vi "Read Joystick.vi"(8 "Joystick Deadbanded Value (default of 0.1)":dbl, 11 "Joystick L 1 DevRef":T1) -> (1 "Joystick R 2 X Axis":dbl, 2 "Joystick L 1 Y Axis":dbl, 3 "Joystick L 1 X Axis":dbl)   [LabVIEW 2014]
uses:
  <vilib>/Rock Robotics/WPI/Joystick/WPI_JoystickDevRef.ctl
  <vilib>/Rock Robotics/WPI/Joystick/WPI_JoystickDeviceEnum.ctl
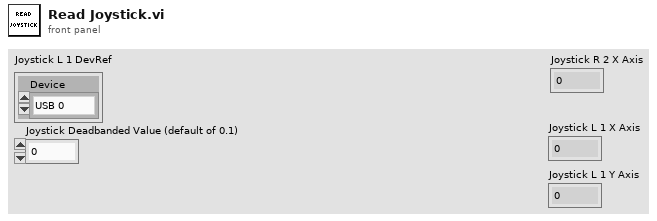
[diagram p1: front panel]
types:
  T1 = typedef "WPI_JoystickDevRef.ctl" = cluster{"Device":T2}
  T2 = typedef "WPI_JoystickDeviceEnum.ctl" = enum16{"USB 0", "USB 1", "USB 2", "USB 3", "USB 4", "USB 5"}
  T3 = cluster{"Buttons[0]":bool, "Buttons[1]":bool, "Buttons[2]":bool, "Buttons[3]":bool, "Buttons[4]":bool, "Buttons[5]":bool, "Buttons[6]":bool, "Buttons[7]":bool, "Buttons[8]":bool}
  T4 = cluster{"Axes[0]":dbl, "Axes[1]":dbl, "Axes[2]":dbl, "Axes[3]":dbl, "Axes[4]":dbl, "Axes[5]":dbl, "Axes[6]":dbl, "Axes[7]":dbl, "Axes[8]":dbl}
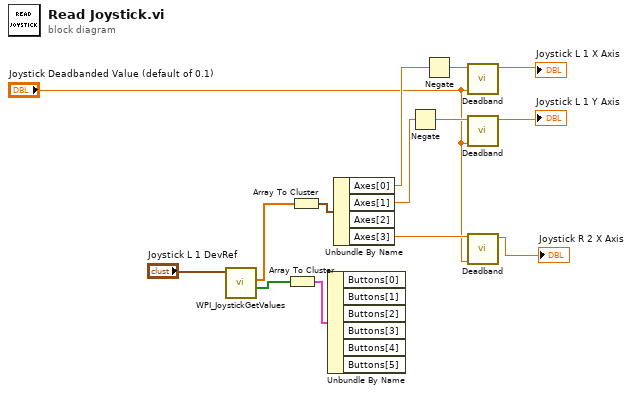
[diagram p0: block diagram]
diagram:
  n1 = call <vilib>:"WPI_JoystickGetValues.vi"("JoystickDevRef"="Joystick L 1 DevRef") -> ("Buttons"=w11:bool[], "Axes"=w13:dbl[])  [unwired: 6 in, 3 out]
  n2 = Array To Cluster(array=w11) -> (cluster=w10:T3)
  n3 = Array To Cluster(array=w13) -> (cluster=w12:T4)
  n4 = Unbundle By Name(w10) -> ()  [unwired: 6 out]
  n5 = Unbundle By Name(w12) -> ("Axes[0]"=w9:dbl, "Axes[1]"=w4:dbl, "Axes[3]"=w3:dbl)  [unwired: 1 out]
  n6 = Negate(x=w4) -> (-x=w5:dbl)
  n7 = Negate(x=w9) -> (-x=w8:dbl)
  n8 = call "Deadband.vi"("Value to Deadband (default of 0.1)"="Joystick Deadbanded Value (default of 0.1)", "Value"=w8) -> ("Deadbanded Value"=→"Joystick L 1 X Axis":dbl)  [unwired: 9 in]
  n9 = call "Deadband.vi"("Value to Deadband (default of 0.1)"="Joystick Deadbanded Value (default of 0.1)", "Value"=w5) -> ("Deadbanded Value"=→"Joystick L 1 Y Axis":dbl)  [unwired: 9 in]
  n10 = call "Deadband.vi"("Value to Deadband (default of 0.1)"="Joystick Deadbanded Value (default of 0.1)", "Value"=w3) -> ("Deadbanded Value"=→"Joystick R 2 X Axis":dbl)  [unwired: 9 in]
